vi "Get Display Text.vi"(8 "error in (no error)":errorcluster, 11 "Element in":refnum<class "Element.lvclass">) -> (0 "error out":errorcluster, 1 "Detail Text":string, 2 "Display Name":string, 3 "Element out":refnum<class "Element.lvclass">)   [LabVIEW 2026, in "VILab.lvlib" / "Element.lvclass"]
uses:
  Element.lvclass
  Element.lvclass/Element.ctl
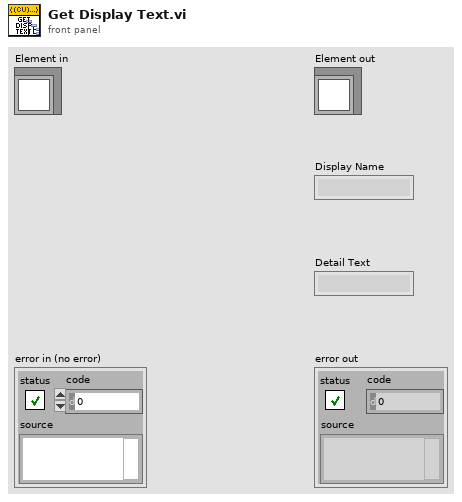
[diagram p1: front panel]
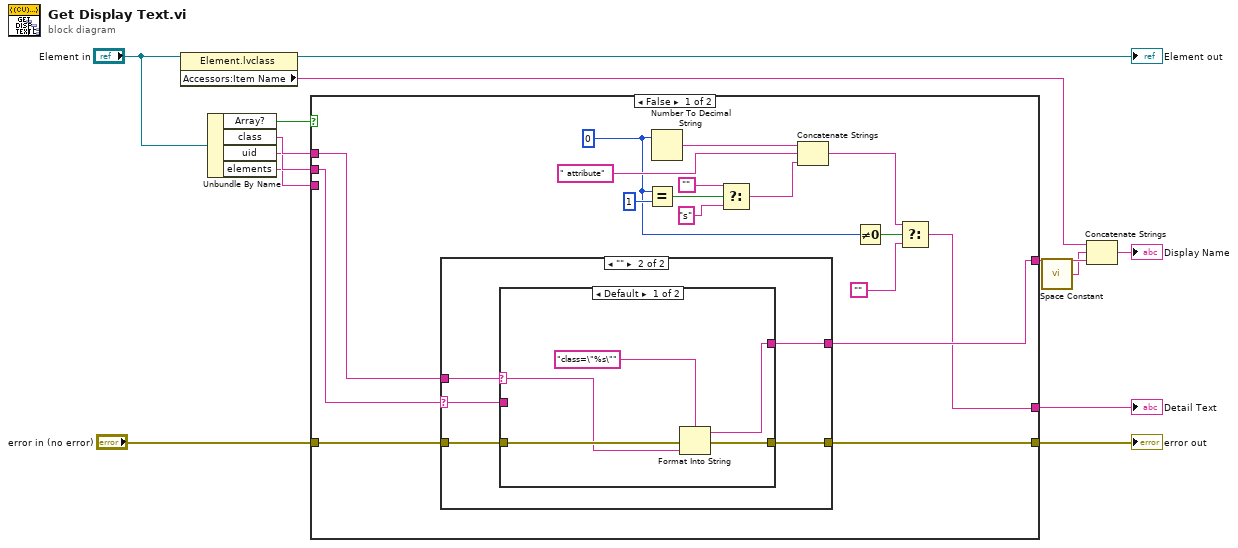
[diagram p0: block diagram]
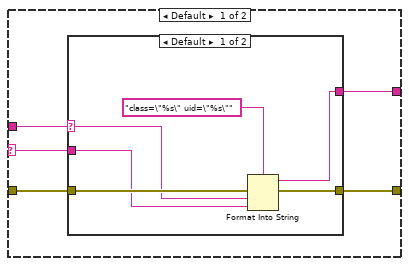
[diagram p2: hidden frame]
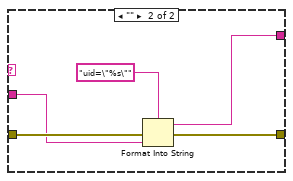
[diagram p3: hidden frame]
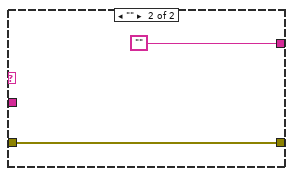
[diagram p4: hidden frame]
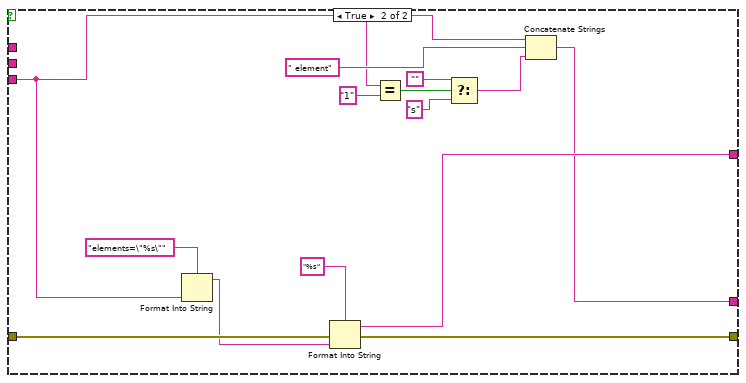
[diagram p5: hidden frame]
diagram:
  n1 = property class="Element.lvclass"(reference="Element in") -> (reference out=→"Element out":refnum<class "Element.lvclass">, "Accessors:Item Name"=w1:string)  [unwired: 1 in, 1 out]
  n2 = Unbundle By Name("Element in") -> ("Array?"=w8:bool, "class"=w11:string, "uid"=w10:string, "elements"=w7:string)
  n3 = case shown="False" w8 {
    tunnel: w11 -> [w15 _]
    tunnel: w10 -> [w16 _]
    tunnel: "error in (no error)" -> [w30 w72]
    tunnel: [w29 w71] -> w12
    tunnel: [w21 w69] -> w4
    tunnel: [w17 w62] -> w9
    tunnel: w7 -> [_ w59]
    frame False {
      w14 = 0 ("number")
      n4 = case shown="\"\"" w16 {
        selector: w16 -> [w31 w47]
        tunnel: w30 -> [w35 w51]
        tunnel: [w34 w50] -> w29
        tunnel: [w33 w49] -> w21
        tunnel: w15 -> [w32 w48]
        frame Default {
          n5 = case shown="Default" w32 {
            selector: w32 -> [w38 _]
            tunnel: w35 -> [w41 w46]
            tunnel: [w40 w45] -> w34
            tunnel: [w36 w42] -> w33
            tunnel: w31 -> [w37 w43]
            frame Default {
              n6 = Format Into String(format string="class=\"%s\" uid=\"%s\"", error in=w41, w38, w37) -> (resulting string=w36:string, error out=w40:errorcluster)  [unwired: 1 in]
            }
            frame "" {
              n7 = Format Into String(format string="uid=\"%s\"", error in=w46, w43) -> (resulting string=w42:string, error out=w45:errorcluster)  [unwired: 1 in]
            }
          }
        }
        frame "" {
          n8 = case shown="Default" w48 {
            selector: w48 -> [w53 _]
            tunnel: w51 -> [w56 w58]
            tunnel: [w55 w58] -> w50
            tunnel: [w52 ""] -> w49
            tunnel: w47 -> [_ _]
            frame Default {
              n9 = Format Into String(format string="class=\"%s\"", error in=w56, w53) -> (resulting string=w52:string, error out=w55:errorcluster)  [unwired: 1 in]
            }
            frame "" {
            }
          }
        }
      }
      n10 = Equal?(x=w14, y=1) -> (x = y?=w26:bool)
      n11 = Number To Decimal String(number=w14) -> (decimal integer string=w28:string)  [unwired: 1 in]
      n12 = Select(t="", s=w26, f="s") -> (s? t:f=w22:string)
      n13 = Concatenate Strings(w28, " attribute", w22) -> (w19:string)
      n14 = Not Equal To 0?(x=w14) -> (x != 0?=w20:bool)
      n15 = Select(t=w19, s=w20, f="") -> (s? t:f=w17:string)
    }
    frame True {
      n16 = Format Into String(format string="elements=\"%s\"", w59) -> (resulting string=w60:string)  [unwired: 2 in, 1 out]
      n17 = Format Into String(format string="%s", error in=w72, w60) -> (resulting string=w69:string, error out=w71:errorcluster)  [unwired: 1 in]
      n18 = Equal?(x=w59, y="1") -> (x = y?=w67:bool)
      n19 = Select(t="", s=w67, f="s") -> (s? t:f=w63:string)
      n20 = Concatenate Strings(w59, " element", w63) -> (w62:string)
    }
  }
  "error out" <- w12
  "Detail Text" <- w9
  n21 = call <vilib>:"Space Constant.vi"() -> ("String"=w2:string)
  n22 = Concatenate Strings(w1, w2, w4) -> (→"Display Name":string)
